vi "Show Array Elements.vi"(6 "Variant in":variant, 7 "Shift Pressed?":bool, 8 "error in (no error)":errorcluster, 10 "QD Combo Box Ref":refnum<vi>, 11 "QD Launch VI Ref":refnum<vi>) -> (0 "error out":errorcluster, 4 "Variant out":variant)   [LabVIEW 2019]
doc: "Changes the selected array(s) to show enough rows/columns to see the empty element just past the end of the array. Works on 1D and 2D arrays.\n\nIf array is 1D, arrays is expanded to show elements in rows if shift is not pressed and in columns if shift is pressed.\n\nDefault Shortcut - [L]"
uses:
  <vilib>/ErrorRing/Error Ring.xnode
panel:
  in  "Undo Name":string="Quick Drop Keyboard Shortcut"
  # "Do not change the connector pane of this VI.\n\nSee the block diagram for directions on how to use this template."
  # "Specify the name of the Undo transaction"
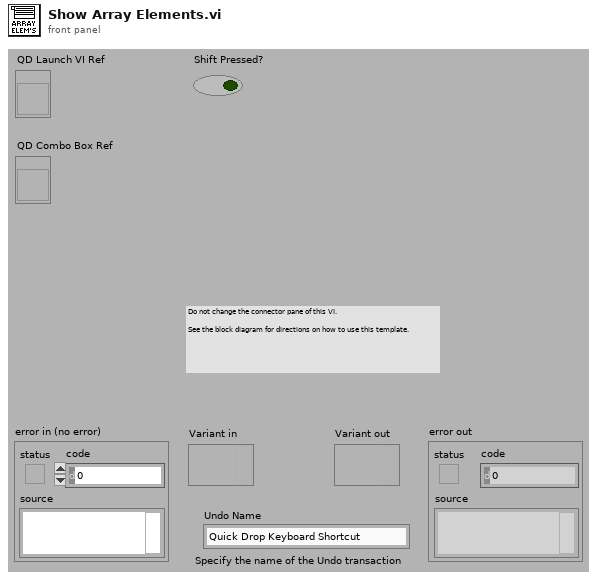
[diagram p1: front panel]
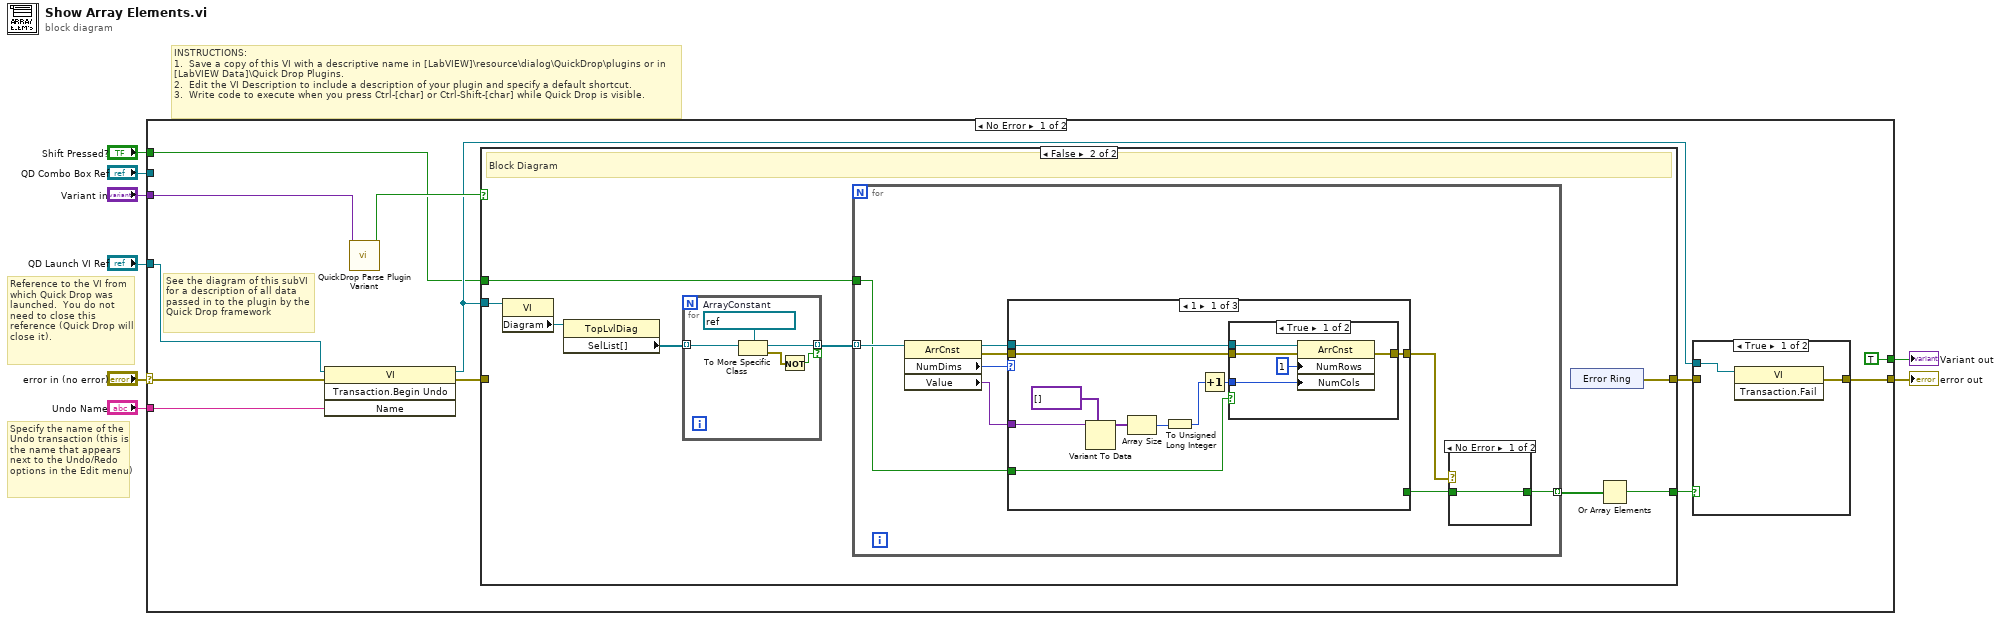
[diagram p0: block diagram]
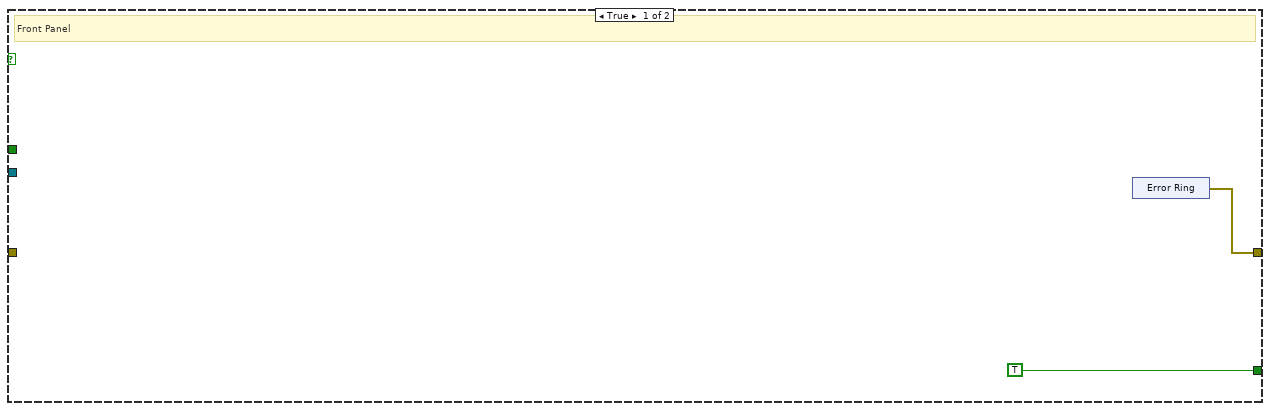
[diagram p2: hidden frame]
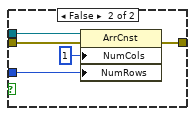
[diagram p3: hidden frame]
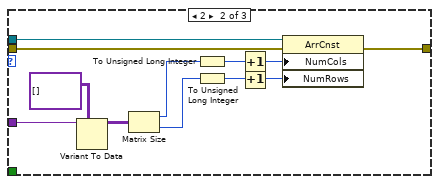
[diagram p4: hidden frame]
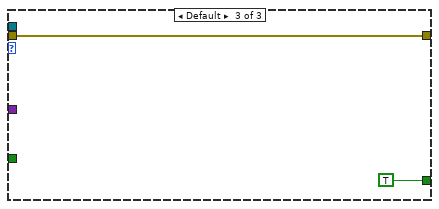
[diagram p5: hidden frame]
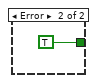
[diagram p6: hidden frame]
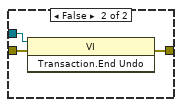
[diagram p7: hidden frame]
diagram:
  # "Specify the name of the Undo transaction (this is the name that appears next to the Undo/Redo options in the Edit menu)"
  # "Reference to the VI from which Quick Drop was launched.  You do not need to close this reference (Quick Drop will close it)."
  # "INSTRUCTIONS:\n1.  Save a copy of this VI with a descriptive name in [LabVIEW]\\resource\\dialog\\QuickDrop\\plugins or in [LabVIEW Data]\\Quick Drop Plugins.\n2.  Edit the VI Description to include a description of your plugin and specify a default shortcut. \n3.  Write code to execute when you press Ctrl-[char] or Ctrl-Shift-[char] while Quick Drop is visible."
  n1 = case shown="No Error" "error in (no error)" {
    selector: "error in (no error)" -> [w19 w88]
    tunnel: [w14 w88] -> w7
    tunnel: "QD Launch VI Ref" -> [w18 _]
    tunnel: "Shift Pressed?" -> [w11 _]
    tunnel: "QD Combo Box Ref" -> [_ _]
    tunnel: "Variant in" -> [w20 _]
    tunnel: "Undo Name" -> [w17 _]
    tunnel: [TRUE _] -> w1
    frame No Error {
      # "See the diagram of this subVI for a description of all data passed in to the plugin by the Quick Drop framework"
      n2 = invoke class="VI" method="Transaction.Begin Undo"(reference=w18, error in=w19, "Name"=w17) -> (reference out=w13:refnum<vi>, error out=w12:errorcluster)  [unwired: 1 in, 2 out]
      n3 = call <vilib>:"QuickDrop Parse Plugin Variant.vi"("QDKS Variant in"=w20) -> ("QD Launch VI Panel?"=w15:bool)  [unwired: 12 in, 2 out]
      n4 = case shown="False" w15 {
        tunnel: w12 -> [_ _]
        tunnel: w13 -> [_ w30]
        tunnel: w11 -> [_ w29]
        tunnel: [w22 w31] -> w10
        tunnel: [TRUE w24] -> w9
        frame True {
          # "Front Panel"
          n5 = xnode "Error Ring"() -> ("error out"=w22:errorcluster)
        }
        frame False {
          # "Block Diagram"
          n6 = property class="VI"(reference=w30) -> ("Diagram"=w25:refnum<vi>)  [unwired: 1 in, 2 out]
          n7 = property class="TopLvlDiag"(reference=w25) -> ("SelList[]"=w27:refnum<vi>[])  [unwired: 1 in, 2 out]
          n8 = for {
            tunnel: w27 -> [w32] mode=indexing
            tunnel: [w35] -> w26 mode=indexing if=w33
            w36 = refnum<vi> refnum  # ArrayConstant
            n9 = To More Specific Class(target class=w36, reference=w32) -> (specific class reference=w35:refnum<vi>, error out=w34:errorcluster)  [unwired: 1 in]
            n10 = Not(x=w34) -> (.not. x?=w33:bool)
          }
          n11 = for {
            tunnel: w29 -> [w40]
            tunnel: w26 -> [w45] mode=indexing
            tunnel: [w44] -> w28 mode=indexing
            n12 = property class="ArrCnst"(reference=w45) -> (reference out=w38:refnum<vi>, error out=w37:errorcluster, "NumDims"=w43:u32, "Value"=w42:variant)  [unwired: 1 in]
            n13 = case shown="1" w43 {
              tunnel: w42 -> [w54 w77 _]
              tunnel: [_ _ TRUE] -> w41
              tunnel: w40 -> [w50 _ _]
              tunnel: [w51 w72 w78] -> w39
              tunnel: w38 -> [w49 w74 _]
              tunnel: w37 -> [w48 w73 w78]
              frame 1 {
                n14 = Variant To Data(type=variant[] [], Variant=w54) -> (data=w53:variant[])  [unwired: 1 in, 1 out]
                n15 = Array Size(array=w53) -> (size(s)=w52:i32)
                n16 = To Unsigned Long Integer(number=w52) -> (unsigned 32bit integer=w47:u32)
                n17 = Increment(x=w47) -> (x+1=w46:u32)
                n18 = case shown="True" w50 {
                  tunnel: w46 -> [w60 w62]
                  tunnel: [w59 w65] -> w51
                  tunnel: w49 -> [w58 w64]
                  tunnel: w48 -> [w57 w63]
                  frame True {
                    n19 = property class="ArrCnst"(reference=w58, error in=w57, "NumRows"=u32 1 ("Number of Rows"), "NumCols"=w60) -> (error out=w59:errorcluster)  [unwired: 1 out]
                  }
                  frame False {
                    n20 = property class="ArrCnst"(reference=w64, error in=w63, "NumCols"=u32 1 ("Number of Columns"), "NumRows"=w62) -> (error out=w65:errorcluster)  [unwired: 1 out]
                  }
                }
              }
              frame 2 {
                n21 = Variant To Data(type=variant[][] [], Variant=w77) -> (data=w75:variant[][])  [unwired: 1 in, 1 out]
                n22 = Matrix Size(0:w75) -> (1:w71:i32, 2:w70:i32)
                n23 = To Unsigned Long Integer(number=w71) -> (unsigned 32bit integer=w69:u32)
                n24 = To Unsigned Long Integer(number=w70) -> (unsigned 32bit integer=w68:u32)
                n25 = Increment(x=w69) -> (x+1=w67:u32)
                n26 = Increment(x=w68) -> (x+1=w66:u32)
                n27 = property class="ArrCnst"(reference=w74, error in=w73, "NumCols"=w67, "NumRows"=w66) -> (error out=w72:errorcluster)  [unwired: 1 out]
              }
              frame Default {
              }
            }
            n28 = case shown="No Error" w39 {
              tunnel: [w80 TRUE] -> w44
              tunnel: w41 -> [w80 _]
              frame No Error {
              }
              frame Error {
              }
            }
          }
          n29 = xnode "Error Ring"() -> ("error out"=w31:errorcluster)
          n30 = Or Array Elements(Boolean array=w28) -> (logical OR=w24:bool)
        }
      }
      n31 = case shown="True" w9 {
        tunnel: w13 -> [w83 w86]
        tunnel: [w84 w87] -> w14
        tunnel: w10 -> [_ w85]
        frame True {
          n32 = invoke class="VI" method="Transaction.Fail"(reference=w83) -> (error out=w84:errorcluster)  [unwired: 2 in, 2 out]
        }
        frame False {
          n33 = invoke class="VI" method="Transaction.End Undo"(reference=w86, error in=w85) -> (error out=w87:errorcluster)  [unwired: 1 in, 2 out]
        }
      }
    }
    frame Error {
    }
  }
  "error out" <- w7
  "Variant out" <- w1
